vi "Teleop.vi"(10 "Match Info":T1={"Autonomous Elapsed Seconds"=0.0, "TeleOp Elapsed Seconds"=0.0, "Disabled Elapsed Seconds"=0.0, "Visited Autonomous"=FALSE, "Visited TeleOp"=FALSE, "Visited Disabled"=FALSE, "Autonomous Settings"={"Autonomous Style"=enum."Independent", "VI Refnum"=refnum}}, 11 "Call Context":T2) -> ()   [LabVIEW 2018]
doc: "This VI is called for each TeleOp packet received from the DS where the robot is not disabled. It is often used to read from the joysticks and update I/O or to update setpoints for timed control loops. It should complete and return within 20 milliseconds or it may miss DS packets."
uses:
  <vilib>/Rock Robotics/WPI/DriverStation/WPI_DriverStationDerivedRobotMode.ctl
  <vilib>/Rock Robotics/WPI/DriverStation/WPI_DriverStationMatch Info.ctl
  <vilib>/Rock Robotics/WPI/Solenoid/WPI_SolenoidValue.ctl
  Robot Global Data.vi
  <vilib>/Rock Robotics/WPI/Solenoid/WPI_SolenoidSetEnum.vi
  <vilib>/Rock Robotics/Network Tables/NT Write Number.vi
  <vilib>/Rock Robotics/WPI/Utilities/WPI_GetSetVariantRefNum.vi
  <vilib>/Rock Robotics/Network Tables/NT Write Numeric Array.vi
  <vilib>/Rock Robotics/Network Tables/NT Write Boolean Array.vi
  <vilib>/Rock Robotics/Network Tables/NT Read Boolean.vi
  <vilib>/Rock Robotics/Network Tables/NT Read Number.vi
panel:
  out "Sample Slider 0":dbl(slide) scale=0.0..5.0
  out "Sample Boolean 1":bool
  out "Sample Boolean 0":bool
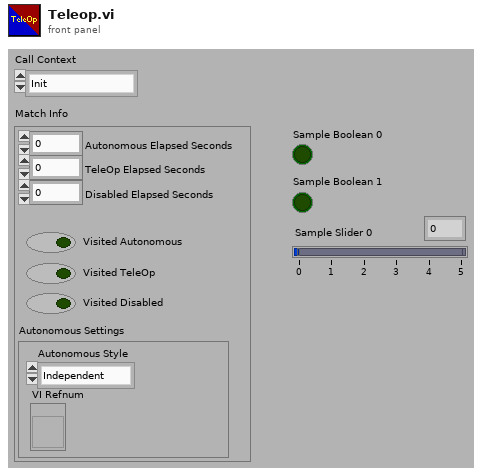
[diagram p1: front panel]
types:
  T1 = typedef "WPI_DriverStationMatch Info.ctl" = cluster{"Autonomous Elapsed Seconds":dbl, "TeleOp Elapsed Seconds":dbl, "Disabled Elapsed Seconds":dbl, "Visited Autonomous":bool, "Visited TeleOp":bool, "Visited Disabled":bool, "Autonomous Settings":cluster{"Autonomous Style":enum16{"Iterative", "Independent"}, "VI Refnum":refnum<vi>}}
  T2 = typedef "WPI_DriverStationDerivedRobotMode.ctl" = enum16{"Init", "Execute", "Stop"}
  T3 = typedef "WPI_RobotDriveDevRef.ctl" = cluster{"DevStatus":errorcluster, "Motors[]":T4[], "Square Inputs":bool, "Max Output":dbl}
  T4 = typedef "WPI_MotorControlDeviceRef.ctl" = cluster{"DeviceStatus":errorcluster, "Type":T5, "PWM":cluster{"PWM Channel":T6, "DeadBand":T7}, "CAN":cluster{"Device Number":u8, "SetOutput VI Ref":variant, "GetOutput VI Ref":variant, "Enable VI Ref":variant, "Disable VI Ref":variant, "Data":variant}, "Invert":bool, "DIO PWM":cluster{"PWM \"Enable\" Channel":T6, "DIOChannel":T8, "PWM Rate":dbl}}
  T5 = typedef "WPI_MotorControlType.ctl" = enum16{"PWM", "CAN", "DIO PWM"}
  T6 = typedef "FPGA_DIOPWMChannel.ctl" = enum8{"PWM 0", "PWM 1", "PWM 2", "PWM 3", "PWM 4", "PWM 5", "PWM 6", "PWM 7", "PWM 8", "PWM 9", "PWM MXP 0", "PWM MXP 1", "PWM MXP 2", "PWM MXP 3", "PWM MXP 4", "PWM MXP 5", "PWM MXP 6", "PWM MXP 7", "PWM MXP 8", "PWM MXP 9", "Invalid"}
  T7 = typedef "WPI_PWMDeadband.ctl" = cluster{"Name":string, "maxPositivePwm":i32, "minPositivePwm":i32, "centerPwm":i32, "maxNegativePwm":i32, "minNegativePwm":i32, "angularRange":u16}
  T8 = typedef "FPGA_DIOChannel.ctl" = enum8{"DIO 0", "DIO 1", "DIO 2", "DIO 3", "DIO 4", "DIO 5", "DIO 6", "DIO 7", "DIO 8", "DIO 9", "DIO MXP 0", "DIO MXP 1", "DIO MXP 2", "DIO MXP 3", "DIO MXP 4", "DIO MXP 5", "DIO MXP 6", "DIO MXP 7", "DIO MXP 8", "DIO MXP 9", "DIO MXP 10", "DIO MXP 11", "DIO MXP 12", "DIO MXP 13", "DIO MXP 14", "DIO MXP 15", "SPI Port CS1", "SPI Port CS2", "SPI Port CS3", "SPI Port MISO", "SPI Port MOSI", "Invalid"}
  T9 = typedef "WPI_SolenoidDevRef.ctl" = cluster{"DevStatus":errorcluster, "Pneumatics Control Module":u8, "Forward Solenoid Channel":T10, "Reverse Solenoid Channel":T10}
  T10 = typedef "WPI_SolenoidChannel.ctl" = enum8{"Solenoid 0", "Solenoid 1", "Solenoid 2", "Solenoid 3", "Solenoid 4", "Solenoid 5", "Solenoid 6", "Solenoid 7", "Invalid"}
  T11 = typedef "WPI_SolenoidValue.ctl" = enum16{"Off", "On", "Forward", "Reverse"}
  T12 = typedef "WPI_JoystickDevRef.ctl" = cluster{"Device":T13}
  T13 = typedef "WPI_JoystickDeviceEnum.ctl" = enum16{"USB 0", "USB 1", "USB 2", "USB 3", "USB 4", "USB 5"}
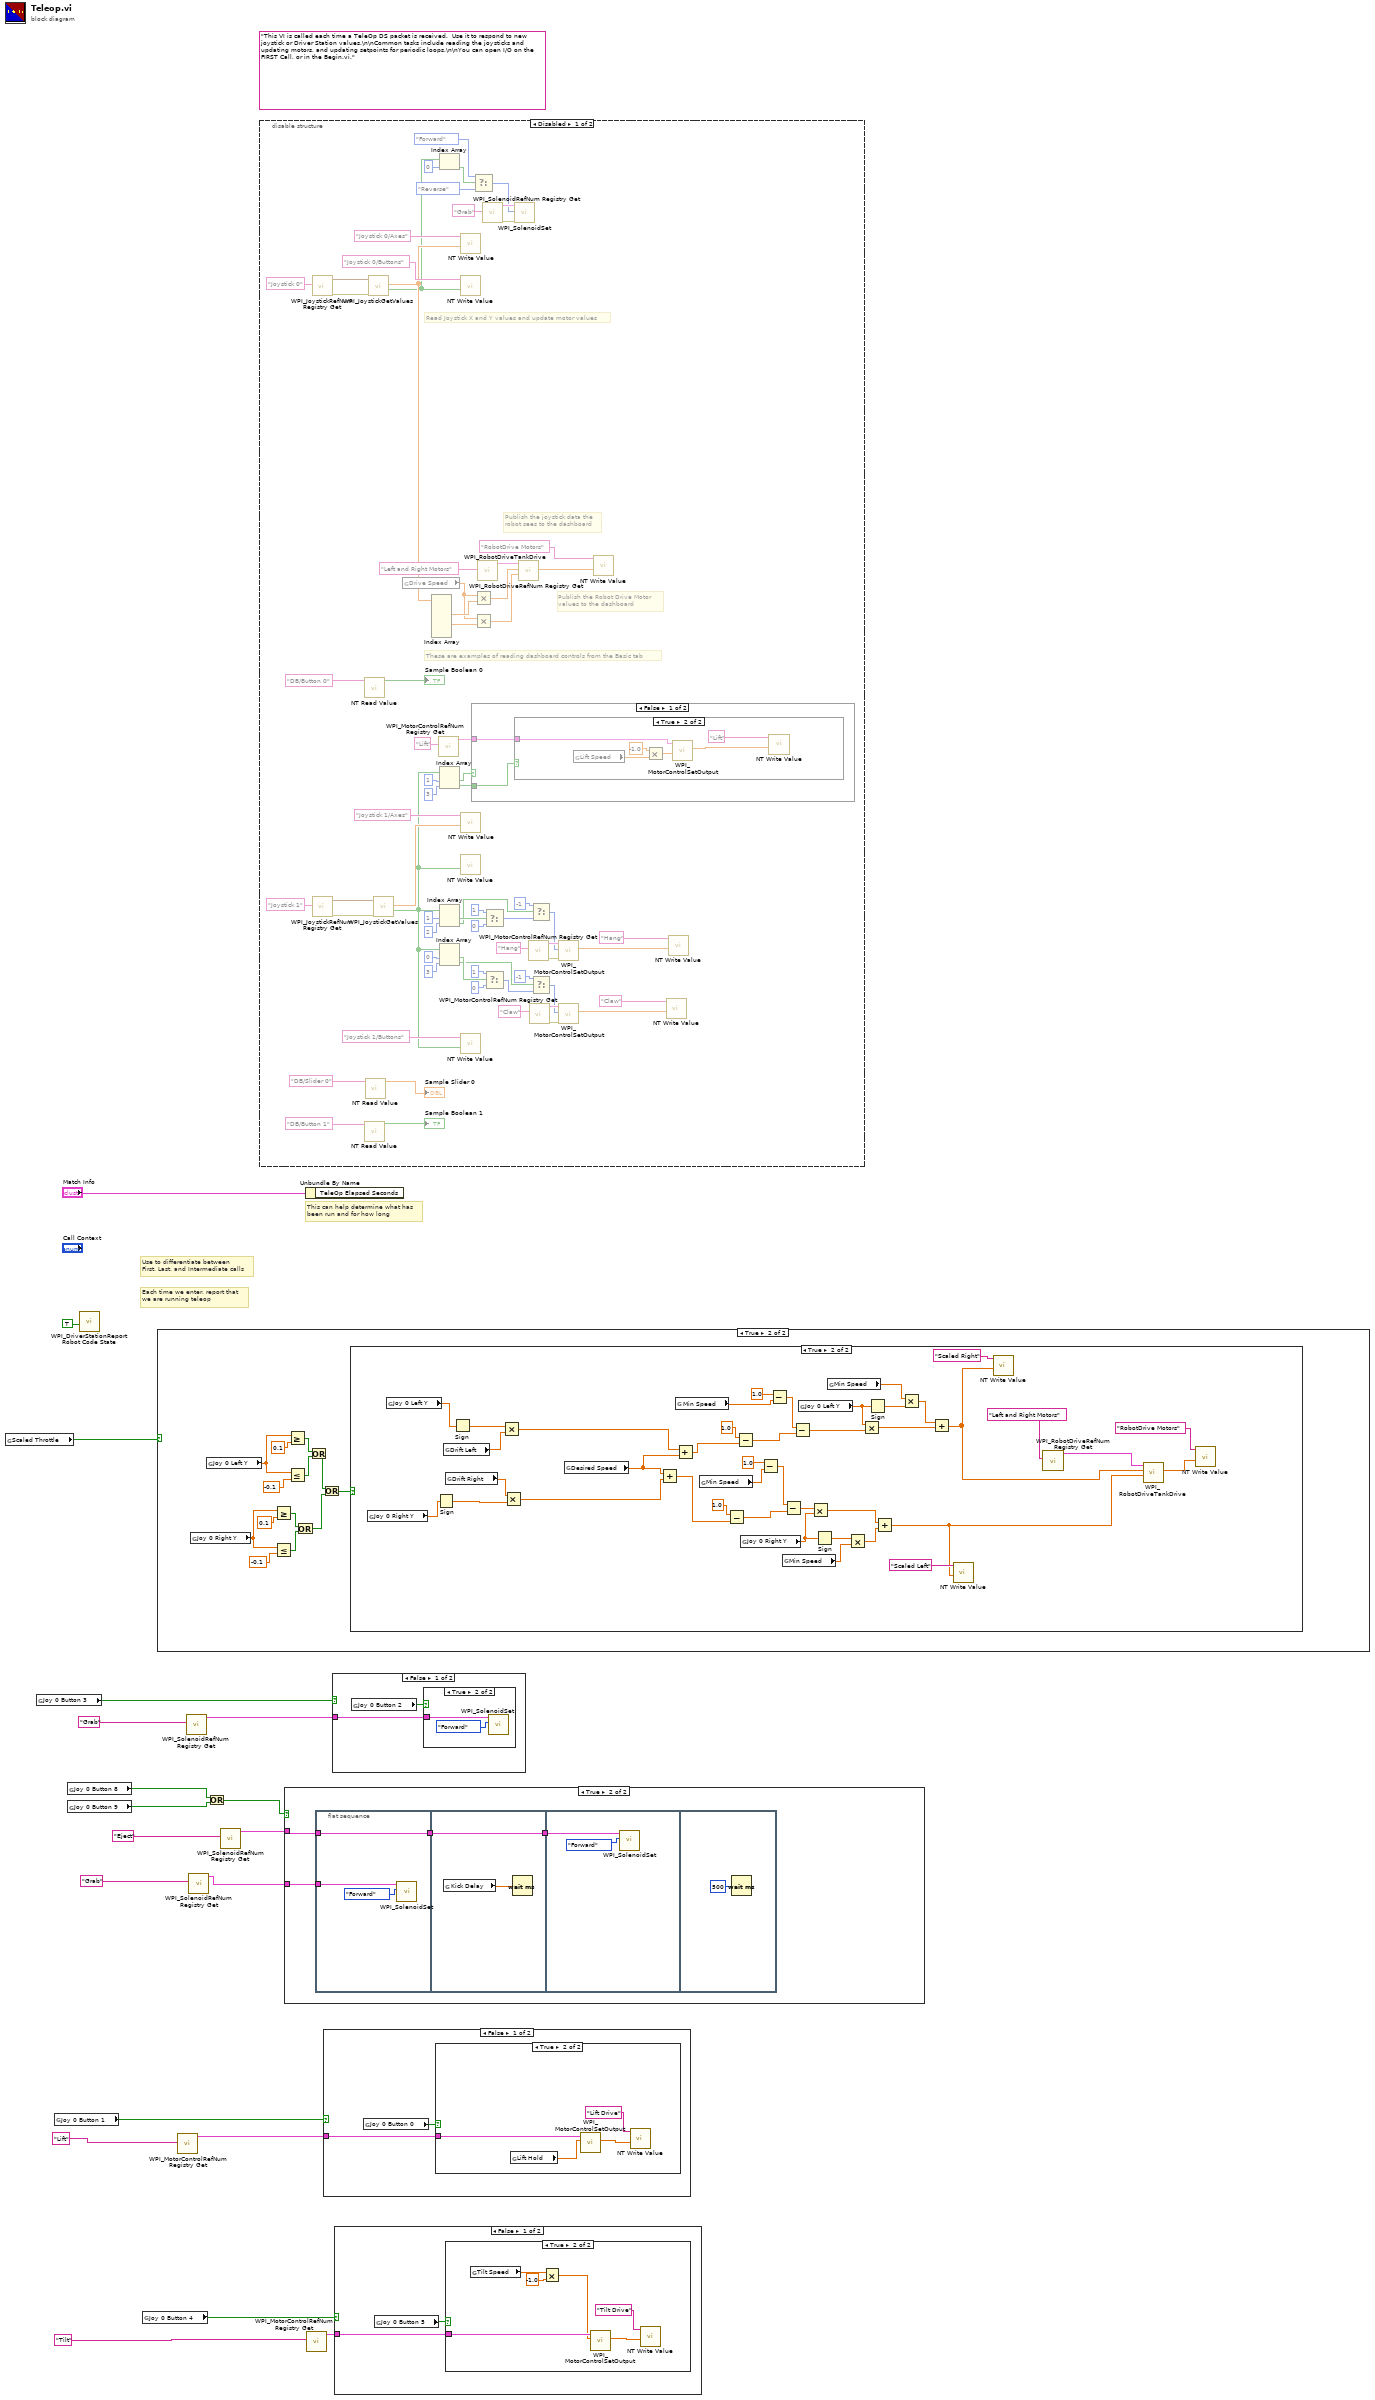
[diagram p0: block diagram]
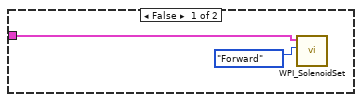
[diagram p2: hidden frame]
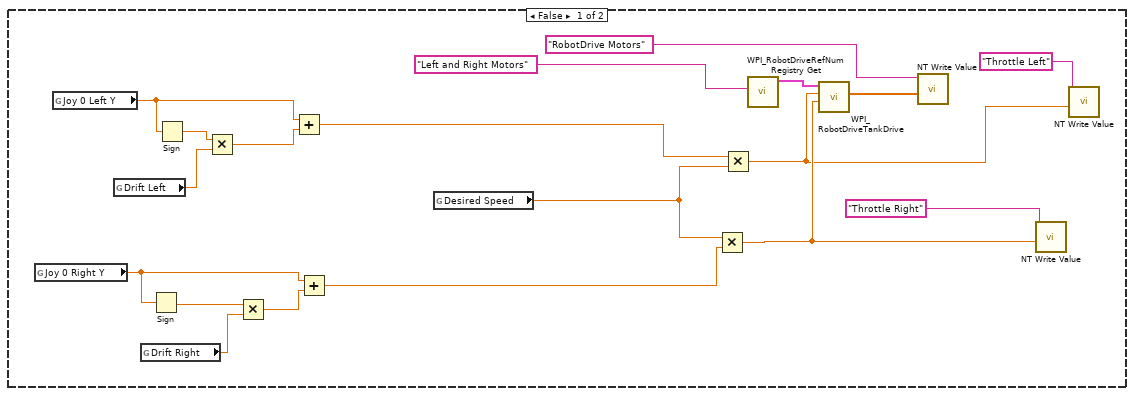
[diagram p3: hidden frame]
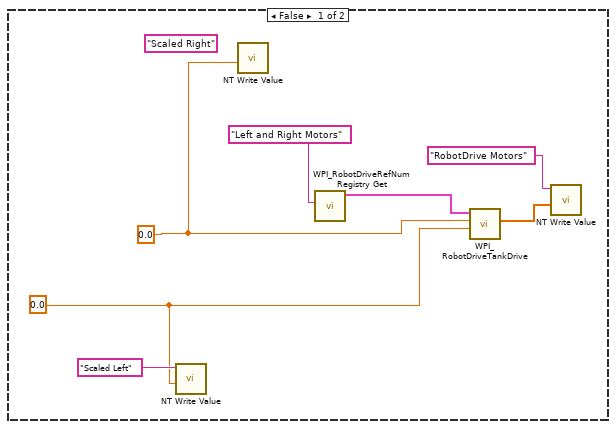
[diagram p4: hidden frame]
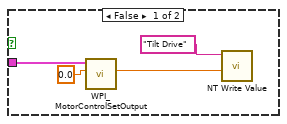
[diagram p5: hidden frame]
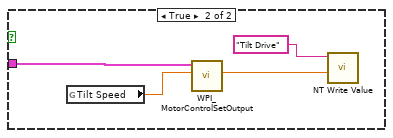
[diagram p6: hidden frame]
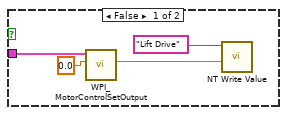
[diagram p7: hidden frame]
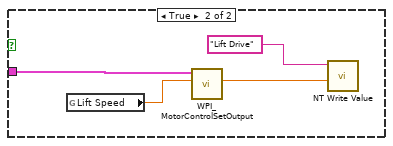
[diagram p8: hidden frame]
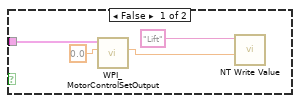
[diagram p9: hidden frame]
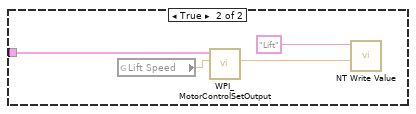
[diagram p10: hidden frame]
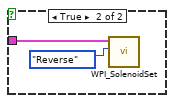
[diagram p13: hidden frame]
diagram:
  (unwired) "This VI is called each time a TeleOp DS packet is received.  Use it to respond to new joystick or Driver Station values.\n\nCommon tasks include reading the joysticks and updating motors, and updating setpoints for periodic loops.\n\nYou can open I/O on the FIRST Call, or in the Begin.vi."
  # "Each time we enter, report that\nwe are running teleop"
  # "Use to differentiate between\nFirst, Last, and Intermediate calls"
  # "This can help determine what has\nbeen run and for how long"
  n1 = global read "Robot Global Data.vi" "Scaled Throttle"() -> (w8:bool)
  n2 = global read "Robot Global Data.vi" "Joy 0 Button 3"() -> (w15:bool)
  n3 = global read "Robot Global Data.vi" "Joy 0 Button 1"() -> (w13:bool)
  n4 = global read "Robot Global Data.vi" "Joy 0 Button 8"() -> (w3:bool)
  n5 = global read "Robot Global Data.vi" "Joy 0 Button 9"() -> (w2:bool)
  n6 = call <vilib>:"WPI_DriverStationReport Robot Code State.vi"("TeleOp"=TRUE ("Autonomous")) -> ()  [unwired: 10 in, 1 out]
  n7 = global read "Robot Global Data.vi" "Joy 0 Button 4"() -> (w10:bool)
  n8 = case shown="True" w8 {
    frame False {
      n9 = global read "Robot Global Data.vi" "Joy 0 Right Y"() -> (w27:dbl)
      n10 = global read "Robot Global Data.vi" "Joy 0 Left Y"() -> (w20:dbl)
      n11 = global read "Robot Global Data.vi" "Drift Left"() -> (w22:dbl)
      n12 = global read "Robot Global Data.vi" "Drift Right"() -> (w24:dbl)
      n13 = Sign(1:w27) -> (0:w25:dbl)
      n14 = Sign(1:w20) -> (0:w21:dbl)
      n15 = Multiply(x=w21, y=w22) -> (x*y=w23:dbl)
      n16 = Multiply(x=w25, y=w24) -> (x*y=w26:dbl)
      n17 = Add(x=w20, y=w23) -> (x+y=w28:dbl)
      n18 = Add(x=w27, y=w26) -> (x+y=w29:dbl)
      n19 = global read "Robot Global Data.vi" "Desired Speed"() -> (w30:dbl)
      n20 = Multiply(x=w30, y=w29) -> (x*y=w32:dbl)
      n21 = Multiply(x=w28, y=w30) -> (x*y=w31:dbl)
      n22 = call <vilib>:"WPI_RobotDriveRefNum Registry Get.vi"("refnum name"="Left and Right Motors") -> ("RobotDriveDevRef"=w35:T3)  [unwired: 1 in, 9 out]
      n23 = call <vilib>:"WPI_RobotDriveTankDrive.vi"("Right axis value"=w32, "Left axis value"=w31, "RobotDriveDevRef"=w35) -> ("Motor Values"=w36:dbl[])  [unwired: 6 in, 2 out]
      n24 = call-poly <vilib>:"NT Write Value.vi"("Numeric Array"=w36, "Name"="RobotDrive Motors") -> ()  [unwired: 9 in, 1 out]
      n25 = call-poly <vilib>:"NT Write Value.vi"("Numeric"=w32, "Name"="Throttle Right") -> ()  [unwired: 9 in, 1 out]
      n26 = call-poly <vilib>:"NT Write Value.vi"("Numeric"=w31, "Name"="Throttle Left") -> ()  [unwired: 9 in, 1 out]
    }
    frame True {
      n27 = global read "Robot Global Data.vi" "Joy 0 Right Y"() -> (w43:dbl)
      n28 = global read "Robot Global Data.vi" "Joy 0 Left Y"() -> (w50:dbl)
      n29 = Greater Or Equal?(x=w43, y=0.1) -> (x >= y?=w41:bool)
      n30 = Less Or Equal?(x=w43, y=-0.1) -> (x <= y?=w40:bool)
      n31 = Greater Or Equal?(x=w50, y=0.1) -> (x >= y?=w48:bool)
      n32 = Less Or Equal?(x=w50, y=-0.1) -> (x <= y?=w47:bool)
      n33 = Or(x=w41, y=w40) -> (x .or. y?=w39:bool)
      n34 = Or(x=w48, y=w47) -> (x .or. y?=w45:bool)
      n35 = Or(x=w45, y=w39) -> (x .or. y?=w46:bool)
      n36 = case shown="True" w46 {
        frame False {
          w52 = 0.0 ("Numeric")
          w53 = 0.0 ("Numeric")
          (unwired) "Scaled Right" ("Name")
          n37 = call-poly <vilib>:"NT Write Value.vi"("Numeric"=w53, "Name"="Scaled Left") -> ()  [unwired: 9 in, 1 out]
          n38 = call-poly <vilib>:"NT Write Value.vi"("Numeric"=w52) -> ()  [unwired: 10 in, 1 out]
          n39 = call <vilib>:"WPI_RobotDriveRefNum Registry Get.vi"("refnum name"="Left and Right Motors") -> ("RobotDriveDevRef"=w55:T3)  [unwired: 1 in, 9 out]
          n40 = call <vilib>:"WPI_RobotDriveTankDrive.vi"("Right axis value"=w53, "Left axis value"=w52, "RobotDriveDevRef"=w55) -> ("Motor Values"=w56:dbl[])  [unwired: 6 in, 2 out]
          n41 = call-poly <vilib>:"NT Write Value.vi"("Numeric Array"=w56, "Name"="RobotDrive Motors") -> ()  [unwired: 9 in, 1 out]
        }
        frame True {
          n42 = global read "Robot Global Data.vi" "Joy 0 Right Y"() -> (w94:dbl)
          n43 = global read "Robot Global Data.vi" "Joy 0 Left Y"() -> (w93:dbl)
          n44 = Sign(1:w94) -> (0:w89:dbl)
          n45 = global read "Robot Global Data.vi" "Drift Left"() -> (w91:dbl)
          n46 = global read "Robot Global Data.vi" "Drift Right"() -> (w90:dbl)
          n47 = Sign(1:w93) -> (0:w92:dbl)
          n48 = Multiply(x=w92, y=w91) -> (x*y=w87:dbl)
          n49 = Multiply(x=w90, y=w89) -> (x*y=w88:dbl)
          n50 = global read "Robot Global Data.vi" "Desired Speed"() -> (w95:dbl)
          n51 = Add(x=w95, y=w88) -> (x+y=w80:dbl)
          n52 = Add(x=w87, y=w95) -> (x+y=w74:dbl)
          n53 = global read "Robot Global Data.vi" "Min Speed"() -> (w78:dbl)
          n54 = global read "Robot Global Data.vi" "Min Speed"() -> (w84:dbl)
          n55 = Subtract(x=1.0, y=w80) -> (x-y=w81:dbl)
          n56 = Subtract(x=1.0, y=w74) -> (x-y=w75:dbl)
          n57 = global read "Robot Global Data.vi" "Joy 0 Right Y"() -> (w71:dbl)
          n58 = Subtract(x=1.0, y=w84) -> (x-y=w83:dbl)
          n59 = Subtract(x=1.0, y=w78) -> (x-y=w77:dbl)
          n60 = global read "Robot Global Data.vi" "Min Speed"() -> (w64:dbl)
          n61 = Subtract(x=w83, y=w81) -> (x-y=w73:dbl)
          n62 = Subtract(x=w77, y=w75) -> (x-y=w72:dbl)
          n63 = global read "Robot Global Data.vi" "Joy 0 Left Y"() -> (w70:dbl)
          n64 = Multiply(x=w73, y=w71) -> (x*y=w62:dbl)
          n65 = Sign(1:w71) -> (0:w69:dbl)
          n66 = global read "Robot Global Data.vi" "Min Speed"() -> (w67:dbl)
          n67 = Multiply(x=w69, y=w64) -> (x*y=w63:dbl)
          n68 = Multiply(x=w70, y=w72) -> (x*y=w65:dbl)
          n69 = Sign(1:w70) -> (0:w68:dbl)
          n70 = Add(x=w62, y=w63) -> (x+y=w59:dbl)
          n71 = Multiply(x=w67, y=w68) -> (x*y=w66:dbl)
          n72 = Add(x=w66, y=w65) -> (x+y=w60:dbl)
          n73 = call-poly <vilib>:"NT Write Value.vi"("Numeric"=w59, "Name"="Scaled Left") -> ()  [unwired: 9 in, 1 out]
          n74 = call-poly <vilib>:"NT Write Value.vi"("Numeric"=w60, "Name"="Scaled Right") -> ()  [unwired: 9 in, 1 out]
          n75 = call <vilib>:"WPI_RobotDriveRefNum Registry Get.vi"("refnum name"="Left and Right Motors") -> ("RobotDriveDevRef"=w96:T3)  [unwired: 1 in, 9 out]
          n76 = call <vilib>:"WPI_RobotDriveTankDrive.vi"("Right axis value"=w59, "Left axis value"=w60, "RobotDriveDevRef"=w96) -> ("Motor Values"=w97:dbl[])  [unwired: 6 in, 2 out]
          n77 = call-poly <vilib>:"NT Write Value.vi"("Numeric Array"=w97, "Name"="RobotDrive Motors") -> ()  [unwired: 9 in, 1 out]
        }
      }
    }
  }
  n78 = call <vilib>:"WPI_MotorControlRefNum Registry Get.vi"("refnum name"="Lift") -> ("MotorControlDevRef"=w12:T4)  [unwired: 9 in, 1 out]
  n79 = call <vilib>:"WPI_SolenoidRefNum Registry Get.vi"("refnum name"="Grab") -> ("SolenoidDevRef"=w16:T9)  [unwired: 9 in, 1 out]
  n80 = call <vilib>:"WPI_SolenoidRefNum Registry Get.vi"("refnum name"="Grab") -> ("SolenoidDevRef"=w4:T9)  [unwired: 9 in, 1 out]
  n81 = Or(x=w3, y=w2) -> (x .or. y?=w1:bool)
  n82 = call <vilib>:"WPI_SolenoidRefNum Registry Get.vi"("refnum name"="Eject") -> ("SolenoidDevRef"=w6:T9)  [unwired: 9 in, 1 out]
  n83 = disable-structure shown="Disabled" {
    frame Disabled {
      # "These are examples of reading dashboard controls from the Basic tab"
      # "Publish the Robot Drive Motor\nvalues to the dashboard"
      # "Publish the joystick data the\nrobot sees to the dashboard"
      # "Read Joystick X and Y values and update motor values"
      n84 = call <vilib>:"WPI_JoystickRefNum Registry Get.vi"("refnum name"="Joystick 0") -> ("error out"=w114:errorcluster, "JoystickDevRef"=w168:T12)  [unwired: 1 in, 8 out]
      n85 = call <vilib>:"WPI_JoystickRefNum Registry Get.vi"("refnum name"="Joystick 1") -> ("error out"=w151:errorcluster, "JoystickDevRef"=w156:T12)  [unwired: 9 in]
      n86 = call-poly <vilib>:"NT Read Value.vi"("Name"="DB/Button 0" ("refnum name")) -> ("Boolean"=→"Sample Boolean 0":bool)  [unwired: 9 in, 1 out]
      n87 = call-poly <vilib>:"NT Read Value.vi"("Name"="DB/Button 1" ("refnum name")) -> ("Boolean"=→"Sample Boolean 1":bool)  [unwired: 9 in, 1 out]
      n88 = call-poly <vilib>:"NT Read Value.vi"("Name"="DB/Slider 0" ("refnum name")) -> ("Numeric"=→"Sample Slider 0":dbl)  [unwired: 9 in, 1 out]
      n89 = call <vilib>:"WPI_JoystickGetValues.vi"("error in (no error)"=w114, "JoystickDevRef"=w168) -> ("Buttons"=w115:bool[], "Axes"=w165:dbl[])  [unwired: 5 in, 3 out]
      n90 = call <vilib>:"WPI_JoystickGetValues.vi"("error in (no error)"=w151, "JoystickDevRef"=w156) -> ("Buttons"=w105:bool[], "Axes"=w152:dbl[])  [unwired: 5 in, 3 out]
      n91 = global read "Robot Global Data.vi" "Drive Speed"() -> (w107:dbl)
      n92 = Index Array(array=w165) -> (element #2=w121:dbl, element #4=w106:dbl)  [unwired: 6 in, 4 out]
      n93 = call <vilib>:"WPI_MotorControlRefNum Registry Get.vi"("refnum name"="Lift") -> ("MotorControlDevRef"=w101:T4)  [unwired: 9 in, 1 out]
      n94 = Index Array(array=w115, index=0) -> (element=w111:bool)
      n95 = Index Array(array=w105, index #1=1 ("index"), index #2=3 ("index")) -> (element #1=w102:bool, element #2=w100:bool)
      n96 = Index Array(array=w105, index #1=1, index #2=2) -> (element #1=w132:bool, element #2=w124:bool)
      n97 = Index Array(array=w105, index #1=0, index #2=3) -> (element #1=w145:bool, element #2=w138:bool)
      n98 = call-poly <vilib>:"NT Write Value.vi"("Boolean Array"=w115, "Name"="Joystick 0/Buttons") -> ()  [unwired: 9 in, 1 out]
      n99 = call-poly <vilib>:"NT Write Value.vi"("Boolean Array"=w105) -> ()  [unwired: 10 in, 1 out]
      n100 = call-poly <vilib>:"NT Write Value.vi"("Boolean Array"=w105, "Name"="Joystick 1/Buttons") -> ()  [unwired: 9 in, 1 out]
      n101 = call-poly <vilib>:"NT Write Value.vi"("Numeric Array"=w165, "Name"="Joystick 0/Axes") -> ()  [unwired: 9 in, 1 out]
      n102 = call-poly <vilib>:"NT Write Value.vi"("Numeric Array"=w152, "Name"="Joystick 1/Axes") -> ()  [unwired: 9 in, 1 out]
      n103 = case shown="False" w102 {
        tunnel: w101 -> [w171 w186]
        tunnel: w100 -> [w172 _]
        frame False {
          n104 = case shown="True" w172 {
            tunnel: w171 -> [w173 w180]
            frame False {
              n105 = call <vilib>:"WPI_MotorControlSetOutput.vi"("Output"=0.0, "MotorControlDevRef"=w173) -> ("Motor Output"=w175:dbl)  [unwired: 7 in, 2 out]
              n106 = call-poly <vilib>:"NT Write Value.vi"("Numeric"=w175, "Name"="Lift") -> ()  [unwired: 9 in, 1 out]
            }
            frame True {
              n107 = global read "Robot Global Data.vi" "Lift Speed"() -> (w178:dbl)
              n108 = Multiply(x=-1.0, y=w178) -> (x*y=w179:dbl)
              n109 = call <vilib>:"WPI_MotorControlSetOutput.vi"("options"=w179, "MotorControlDevRef"=w180) -> ("Motor Output"=w181:dbl)  [unwired: 7 in, 2 out]
              n110 = call-poly <vilib>:"NT Write Value.vi"("Numeric"=w181, "Name"="Lift") -> ()  [unwired: 9 in, 1 out]
            }
          }
        }
        frame True {
          n111 = global read "Robot Global Data.vi" "Lift Speed"() -> (w185:dbl)
          n112 = call <vilib>:"WPI_MotorControlSetOutput.vi"("Output"=w185, "MotorControlDevRef"=w186) -> ("Motor Output"=w183:dbl)  [unwired: 7 in, 2 out]
          n113 = call-poly <vilib>:"NT Write Value.vi"("Numeric"=w183, "Name"="Lift") -> ()  [unwired: 9 in, 1 out]
        }
      }
      n114 = Select(t=WPI_SolenoidValue."Forward" ("Value"), s=w111, f=WPI_SolenoidValue."Reverse" ("Value")) -> (s? t:f=w109:T11)
      n115 = Multiply(x=w107, y=w121) -> (x*y=w120:dbl)
      n116 = Multiply(x=w107, y=w106) -> (x*y=w108:dbl)
      n117 = call <vilib>:"WPI_RobotDriveRefNum Registry Get.vi"("refnum name"="Left and Right Motors") -> ("RobotDriveDevRef"=w149:T3)  [unwired: 1 in, 9 out]
      n118 = call <vilib>:"WPI_SolenoidRefNum Registry Get.vi"("refnum name"="Grab") -> ("error out"=w116:errorcluster, "SolenoidDevRef"=w117:T9)  [unwired: 9 in]
      n119 = Select(t=1, s=w132, f=0) -> (s? t:f=w126:i32)
      n120 = Select(t=1, s=w145, f=0) -> (s? t:f=w140:i32)
      n121 = call-poly <vilib>:"WPI_SolenoidSet.vi"("error in (no error)"=w116, "Value"=w109, "SolenoidDevRef"=w117) -> ()  [unwired: 7 in, 2 out]
      n122 = call <vilib>:"WPI_RobotDriveTankDrive.vi"("Right axis value"=w108, "Left axis value"=w120, "RobotDriveDevRef"=w149) -> ("Motor Values"=w150:dbl[])  [unwired: 6 in, 2 out]
      n123 = call <vilib>:"WPI_MotorControlRefNum Registry Get.vi"("refnum name"="Hang") -> ("error out"=w134:errorcluster, "MotorControlDevRef"=w135:T4)  [unwired: 9 in]
      n124 = call <vilib>:"WPI_MotorControlRefNum Registry Get.vi"("refnum name"="Claw") -> ("error out"=w147:errorcluster, "MotorControlDevRef"=w148:T4)  [unwired: 9 in]
      n125 = Select(t=-1, s=w124, f=w126) -> (s? t:f=w129:i32)
      n126 = Select(t=-1, s=w138, f=w140) -> (s? t:f=w110:i32)
      n127 = call <vilib>:"WPI_MotorControlSetOutput.vi"("error in (no error)"=w134, "Output"=w129, "MotorControlDevRef"=w135) -> ("Motor Output"=w123:dbl)  [unwired: 6 in, 2 out]
      n128 = call <vilib>:"WPI_MotorControlSetOutput.vi"("error in (no error)"=w147, "Output"=w110, "MotorControlDevRef"=w148) -> ("Motor Output"=w137:dbl)  [unwired: 6 in, 2 out]
      n129 = call-poly <vilib>:"NT Write Value.vi"("Numeric Array"=w150, "Name"="RobotDrive Motors") -> ()  [unwired: 9 in, 1 out]
      n130 = call-poly <vilib>:"NT Write Value.vi"("Numeric"=w137, "Name"="Claw") -> ()  [unwired: 9 in, 1 out]
      n131 = call-poly <vilib>:"NT Write Value.vi"("Numeric"=w123, "Name"="Hang") -> ()  [unwired: 9 in, 1 out]
    }
    frame Enabled {
    }
  }
  n132 = case shown="True" w1 {
    tunnel: w6 -> [w187 w192]
    tunnel: w4 -> [_ w191]
    frame False {
      n133 = call-poly <vilib>:"WPI_SolenoidSet.vi"("Value"=WPI_SolenoidValue."Forward", "SolenoidDevRef"=w187) -> ()  [unwired: 8 in, 2 out]
    }
    frame True {
      n134 = flat-sequence {
        tunnel: w192 -> [w195]
        tunnel: [w195] -> w190
        tunnel: w191 -> [w193]
        tunnel: w190 -> [w197]
        tunnel: [w197] -> w189
        tunnel: w189 -> [w199]
        frame #0 {
          n135 = call-poly <vilib>:"WPI_SolenoidSet.vi"("Value"=WPI_SolenoidValue."Forward", "SolenoidDevRef"=w193) -> ()  [unwired: 8 in, 2 out]
        }
        frame #1 {
          n136 = global read "Robot Global Data.vi" "Kick Delay"() -> (w196:dbl)
          n137 = Wait (ms)(milliseconds to wait=w196) -> ()  [unwired: 1 out]
        }
        frame #2 {
          n138 = call-poly <vilib>:"WPI_SolenoidSet.vi"("Value"=WPI_SolenoidValue."Forward", "SolenoidDevRef"=w199) -> ()  [unwired: 8 in, 2 out]
        }
        frame #3 {
          n139 = Wait (ms)(milliseconds to wait=u32 500) -> ()  [unwired: 1 out]
        }
      }
    }
  }
  n140 = Unbundle By Name("Match Info") -> ()  [unwired: 1 out]
  n141 = call <vilib>:"WPI_MotorControlRefNum Registry Get.vi"("refnum name"="Tilt") -> ("MotorControlDevRef"=w9:T4)  [unwired: 9 in, 1 out]
  n142 = case shown="False" w13 {
    tunnel: w12 -> [w201 w212]
    frame False {
      n143 = global read "Robot Global Data.vi" "Joy 0 Button 0"() -> (w202:bool)
      n144 = case shown="True" w202 {
        tunnel: w201 -> [w203 w208]
        frame False {
          n145 = call <vilib>:"WPI_MotorControlSetOutput.vi"("Output"=0.0, "MotorControlDevRef"=w203) -> ("Motor Output"=w205:dbl)  [unwired: 7 in, 2 out]
          n146 = call-poly <vilib>:"NT Write Value.vi"("Numeric"=w205, "Name"="Lift Drive") -> ()  [unwired: 9 in, 1 out]
        }
        frame True {
          n147 = global read "Robot Global Data.vi" "Lift Hold"() -> (w207:dbl)
          n148 = call <vilib>:"WPI_MotorControlSetOutput.vi"("Output"=w207, "MotorControlDevRef"=w208) -> ("Motor Output"=w209:dbl)  [unwired: 7 in, 2 out]
          n149 = call-poly <vilib>:"NT Write Value.vi"("Numeric"=w209, "Name"="Lift Drive") -> ()  [unwired: 9 in, 1 out]
        }
      }
    }
    frame True {
      n150 = global read "Robot Global Data.vi" "Lift Speed"() -> (w211:dbl)
      n151 = call <vilib>:"WPI_MotorControlSetOutput.vi"("Output"=w211, "MotorControlDevRef"=w212) -> ("Motor Output"=w213:dbl)  [unwired: 7 in, 2 out]
      n152 = call-poly <vilib>:"NT Write Value.vi"("Numeric"=w213, "Name"="Lift Drive") -> ()  [unwired: 9 in, 1 out]
    }
  }
  n153 = case shown="False" w15 {
    tunnel: w16 -> [w215 w220]
    frame False {
      n154 = global read "Robot Global Data.vi" "Joy 0 Button 2"() -> (w216:bool)
      n155 = case shown="True" w216 {
        tunnel: w215 -> [_ w217]
        frame False {
        }
        frame True {
          n156 = call-poly <vilib>:"WPI_SolenoidSet.vi"("Value"=WPI_SolenoidValue."Forward", "SolenoidDevRef"=w217) -> ()  [unwired: 8 in, 2 out]
        }
      }
    }
    frame True {
      n157 = call-poly <vilib>:"WPI_SolenoidSet.vi"("Value"=WPI_SolenoidValue."Reverse", "SolenoidDevRef"=w220) -> ()  [unwired: 8 in, 2 out]
    }
  }
  n158 = case shown="False" w10 {
    tunnel: w9 -> [w221 w234]
    frame False {
      n159 = global read "Robot Global Data.vi" "Joy 0 Button 5"() -> (w222:bool)
      n160 = case shown="True" w222 {
        tunnel: w221 -> [w223 w230]
        frame False {
          n161 = call <vilib>:"WPI_MotorControlSetOutput.vi"("Output"=0.0, "MotorControlDevRef"=w223) -> ("Motor Output"=w225:dbl)  [unwired: 7 in, 2 out]
          n162 = call-poly <vilib>:"NT Write Value.vi"("Numeric"=w225, "Name"="Tilt Drive") -> ()  [unwired: 9 in, 1 out]
        }
        frame True {
          n163 = global read "Robot Global Data.vi" "Tilt Speed"() -> (w229:dbl)
          n164 = Multiply(x=w229, y=-1.0) -> (x*y=w227:dbl)
          n165 = call <vilib>:"WPI_MotorControlSetOutput.vi"("Output"=w227, "MotorControlDevRef"=w230) -> ("Motor Output"=w231:dbl)  [unwired: 7 in, 2 out]
          n166 = call-poly <vilib>:"NT Write Value.vi"("Numeric"=w231, "Name"="Tilt Drive") -> ()  [unwired: 9 in, 1 out]
        }
      }
    }
    frame True {
      n167 = global read "Robot Global Data.vi" "Tilt Speed"() -> (w233:dbl)
      n168 = call <vilib>:"WPI_MotorControlSetOutput.vi"("Output"=w233, "MotorControlDevRef"=w234) -> ("Motor Output"=w235:dbl)  [unwired: 7 in, 2 out]
      n169 = call-poly <vilib>:"NT Write Value.vi"("Numeric"=w235, "Name"="Tilt Drive") -> ()  [unwired: 9 in, 1 out]
    }
  }
